vi "soundIn_out.vi"() -> ()   [LabVIEW 2014]
uses:
  <vilib>/sound2/lvsound2.llb/Sound File Info (path).vi
  <vilib>/measure/NI_MAPro.lvlib
  <vilib>/measure/maspectr.llb/FFT Power Spectrum and PSD for 1 Chan.vi
  <vilib>/Math Plots/3D Math Plots/3D Scatter/3D Scatter Datatype/3D Scatter Datatype.lvclass
  <vilib>/Math Plots/3D Math Plots/3D Scatter/3D Scatter Datatype/Public/Plot Helper (Vector).vi
  <vilib>/imath/engines/lvmath2/RunTimeEngine/Managers/WorkSpace/UID Generator.vi
  <vilib>/imath/engines/lvmath2/RunTimeEngine/BuiltInFunctions/length/NIMS_length(GV).vi
  <vilib>/imath/engines/lvmath2/RunTimeEngine/RangeToken/NIMS_Range.vi
  <vilib>/imathl/engines/lvmath/Functions/Error Handling/Create Error.vi
  <vilib>/imath/engines/lvmath2/RunTimeEngine/LocalVariableDefStatement/MC_LocalVariableDefStatement_Display.vi
  <vilib>/imath/engines/lvmath2/RunTimeEngine/RunTimeType/NIMS_RunTimeType_From StrictType (excl LVString).vi
  <vilib>/imath/engines/lvmath2/RunTimeEngine/BuiltInFunctions/ones/NIMS_M=ones(I32).vi
  <vilib>/imath/engines/lvmath2/RunTimeEngine/IndexRead/NIMS M($,S).vi
  <vilib>/imath/engines/lvmath2/RunTimeEngine/RunTimeType/NIMS_RunTimeType_Set Source Original Bool.vi
  <vilib>/imath/engines/lvmath2/RunTimeEngine/Managers/SymbolTable/Clear UID.vi
  <vilib>/imath/engines/lvmath2/RunTimeEngine/NodeEndStatement/NIMS_NodeEndStatement_Output.vi
  <vilib>/imath/engines/lvmath2/RunTimeEngine/ErrorHandling/NIMS_Finalize Error.vi
  <vilib>/sound2/lvsound2.llb/Sound Data Format.ctl
  <vilib>/Math Plots/3D Math Plots/3D Scatter/3D Scatter XCtrl/3D Scatter.xctl
panel:
  out "Time Dependent Power Spectrum":refnum<class "3D Plot Datatype.lvclass">[](xcontrol)
  in  "Play Output":bool
  out "Frequency Power Spectrum":cluster{"f0":dbl, "df":dbl, "magnitude":dbl[]}(graph)={"f0"=0.0, "df"=0.3333333333333333, "magnitude"=array[4500 elements]}
  out "Sound Format: File 2":T1={"sample rate (S/s)"=3000.0, "number of channels"=1, "bits per sample"=16}
  out "Input Audio 2 Waveform":waveform(dbl)(graph)={"t0"=timestamp(0 s since 1904-01-01), "dt"=0.0003333333333333333, "Y"=array[9000 elements]}
  in  "Audio File 2 Path":path=path "C:/Users/jjb22/Documents/GitHub/434_Final_Project/audio_out0.wav"
  in  "Output File Path":path=path "C:/Users/jjb22/Documents/GitHub/434_Final_Project/audio_out1.wav"
  out "Mixed Output Audio Waveform":waveform(dbl)(graph)={"t0"=timestamp(0 s since 1904-01-01), "dt"=0.0003333333333333333, "Y"=array[9000 elements]}
  out "Sound Format: File 1":T1={"sample rate (S/s)"=3000.0, "number of channels"=1, "bits per sample"=16}
  out "Input Audio 1 Waveform":waveform(dbl)(graph)={"t0"=timestamp(0 s since 1904-01-01), "dt"=0.0003333333333333333, "Y"=array[9000 elements]}
  in  "Audio File 1 Path":path=path "C:/Users/jjb22/Documents/GitHub/434_Final_Project/audio_out.wav"
  # "File Name: soundIn_out.vi\nAuthored: Josh Reyes & Josh Borgman\n\nThis VI takes in two audio files and mixes them and normalizes the signal. Optional playback of the mixed output. The power spectrum is computed an ploted below to help the user visualize the audio content."
  # "The plots below use a FFT to compute the power spectrum of the mixed audio signal. The 3D scatter plot displays the power spectrum of 1 second clips  to better visualize the frequency content distribution of the mix signal. The Frequency Power Spectrum displays the power spectrum of the entire waveform."
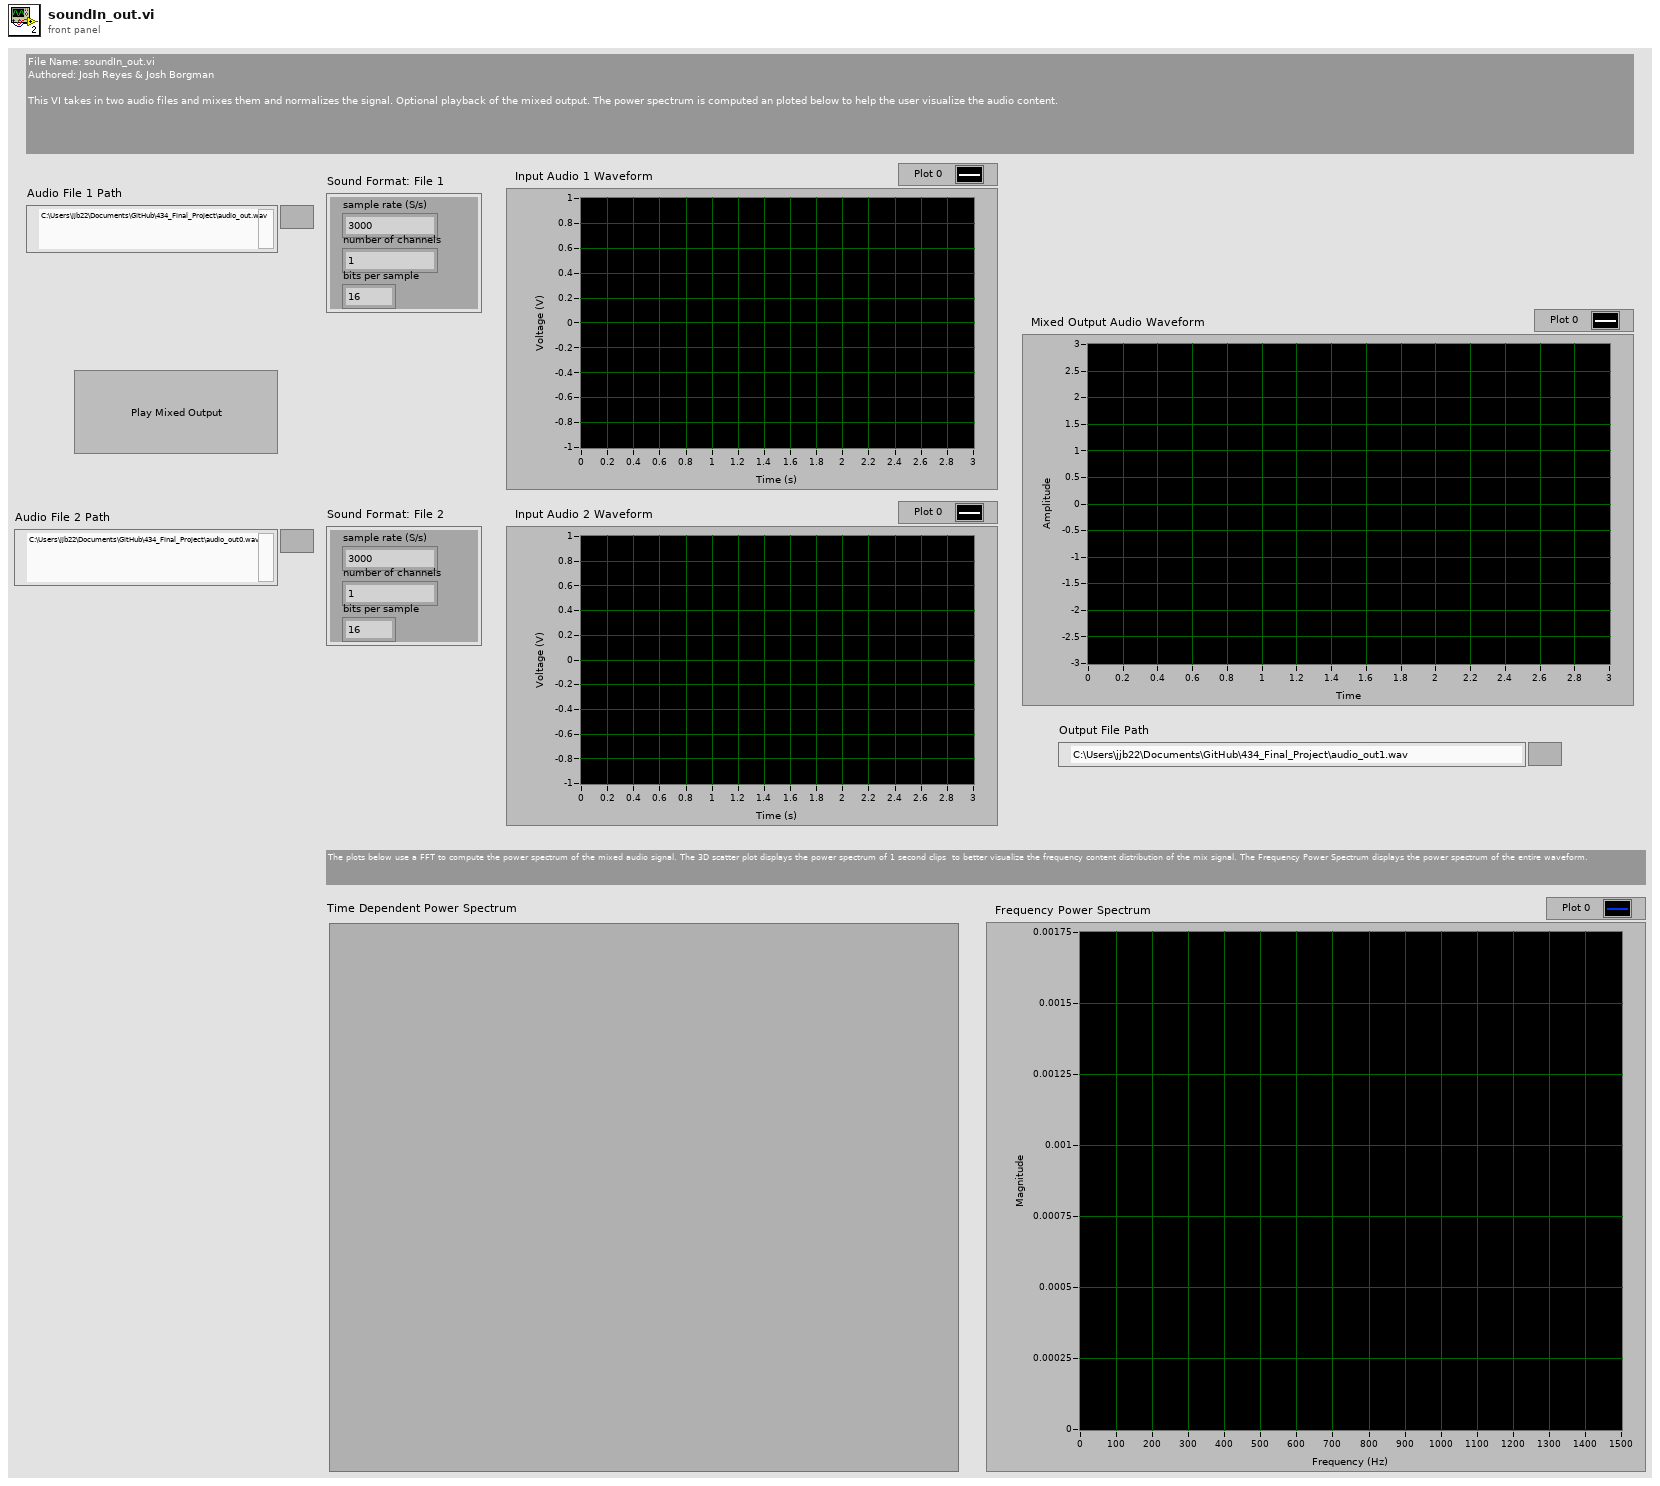
[diagram p1: front panel]
types:
  T1 = typedef "Sound Data Format.ctl" = cluster{"sample rate (S/s)":dbl, "number of channels":i32, "bits per sample":i32}
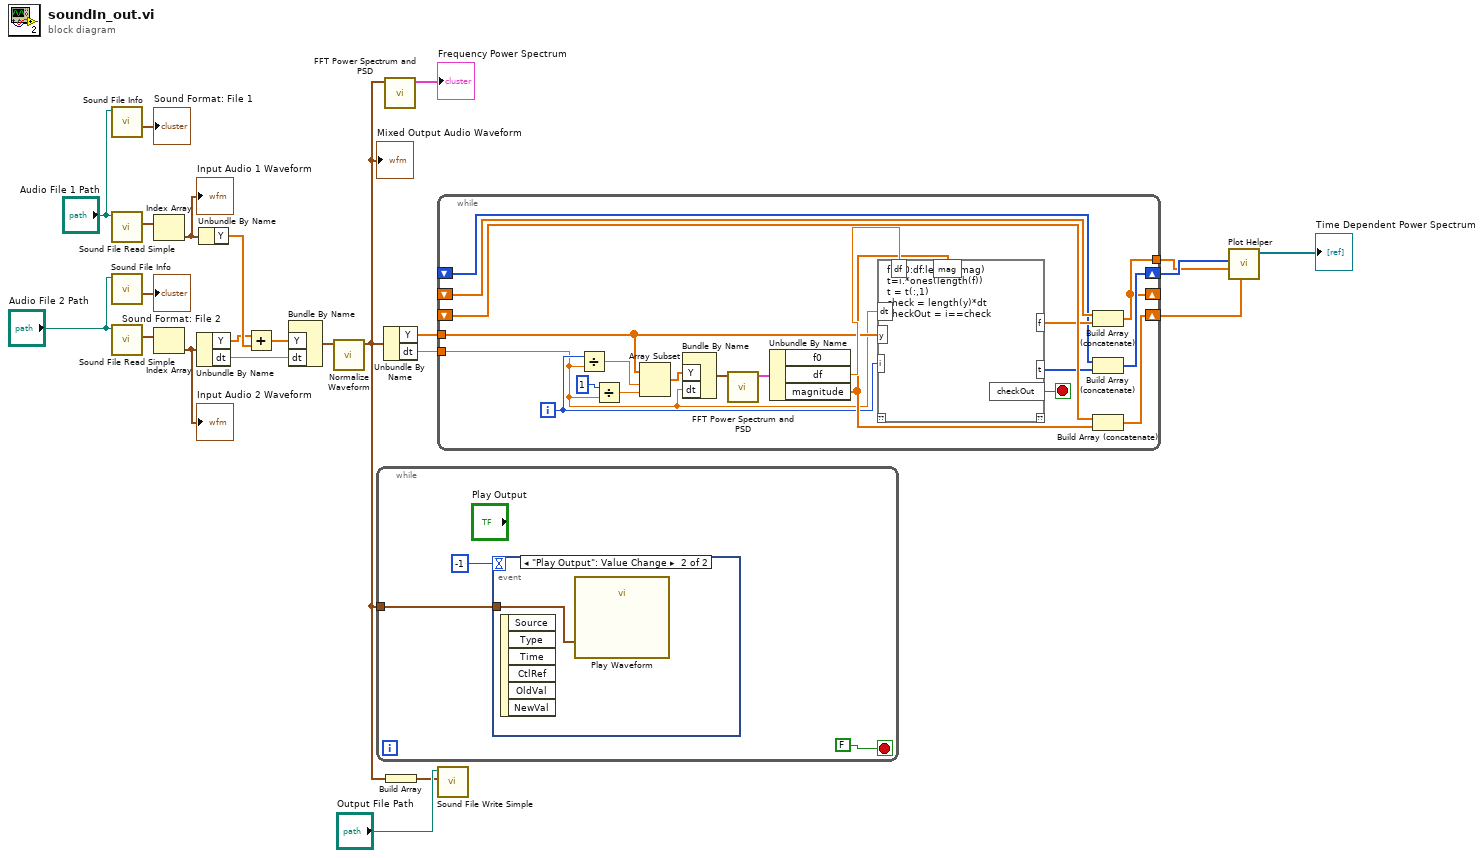
[diagram p0: block diagram]
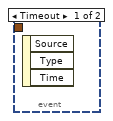
[diagram p2: hidden frame]
diagram:
  n1 = call-poly <vilib>:"Sound File Info.vi"("path"="Audio File 1 Path") -> ("sound format"=→"Sound Format: File 1":T1)  [unwired: 7 in, 3 out]
  n2 = call <vilib>:"Sound File Read Simple.vi"("path"="Audio File 1 Path") -> ("data"=w23:waveform(dbl)[])  [unwired: 7 in, 3 out]
  n3 = call-poly <vilib>:"Sound File Info.vi"("path"="Audio File 2 Path") -> ("sound format"=→"Sound Format: File 2":T1)  [unwired: 7 in, 3 out]
  n4 = call <vilib>:"Sound File Read Simple.vi"("path"="Audio File 2 Path") -> ("data"=w18:waveform(dbl)[])  [unwired: 7 in, 3 out]
  n5 = Index Array(array=w23) -> (element=w22:waveform(dbl))  [unwired: 1 in]
  "Input Audio 1 Waveform" <- w22
  n6 = Index Array(array=w18) -> (element=w17:waveform(dbl))  [unwired: 1 in]
  "Input Audio 2 Waveform" <- w17
  n7 = Unbundle By Name(w17) -> ("Y"=w10:dbl[], "dt"=w9:dbl)
  n8 = Unbundle By Name(w22) -> ("Y"=w13:dbl[])
  n9 = Add(x=w10, y=w13) -> (x+y=w14:dbl[])
  n10 = Bundle By Name("Y"=w14, "dt"=w9) -> (w11:waveform(dbl))  [unwired: 1 in]
  n11 = call <vilib>:"Normalize Waveform.vi"("waveform in"=w11) -> ("normalized waveform"=w7:waveform(dbl))  [unwired: 7 in, 3 out]
  "Mixed Output Audio Waveform" <- w7
  n12 = while {
    tunnel: w7 -> [w25]
    stop <- FALSE stop-if-true
    n13 = event shown="[1] \"Play Output\": Value Change" {
      selector: _ -> [_ _]
      dyn-events: _ -> [_ _]
      timeout: -1 -> [_ _]
      tunnel: w25 -> [_ w27]
      event Timeout {
        n14 = event-data() -> ()  [unwired: 1 in, 3 out]
      }
      event "Play Output": Value Change {
        n15 = event-data() -> ()  [unwired: 1 in, 6 out]
        n16 = call "Play Waveform"("Data"=w27) -> ()  [unwired: 18 in, 1 out]
      }
    }
  }
  n17 = Unbundle By Name(w7) -> ("Y"=w6:dbl[], "dt"=w5:dbl)
  n18 = call-poly <vilib>:"FFT Power Spectrum and PSD.vi"("time signal"=w7) -> ("Power Spectrum / PSD"=→"Frequency Power Spectrum":cluster{"f0":dbl, "df":dbl, "magnitude":dbl[]})  [unwired: 7 in, 3 out]
  n19 = Build Array(w7) -> (w12:waveform(dbl)[])
  n20 = while {
    tunnel: w6 -> [w30]
    tunnel: w5 -> [w29]
    shift-right: [w38] -> w1
    shift-left: _ -> [w40]
    shift-right: [w31] -> _
    shift-left: _ -> [w36]
    shift-right: [w32] -> w3
    shift-left: _ -> [w33]
    tunnel: [w31] -> w2
    i -> [w35]
    stop <- w28 stop-if-true
    n21 = Divide(x=w35, y=w29) -> (x/y=w46:dbl)
    n22 = Divide(x=1, y=w29) -> (x/y=w45:dbl)
    n23 = Array Subset(array=w30, index=w46, length=w45) -> (w43:dbl[])
    n24 = Bundle By Name("Y"=w43, "dt"=w29) -> (w47:waveform(dbl))  [unwired: 1 in]
    n25 = call-poly <vilib>:"FFT Power Spectrum and PSD.vi"("time signal"=w47) -> ("Power Spectrum / PSD"=w42:cluster{"f0":dbl, "df":dbl, "magnitude":dbl[]})  [unwired: 7 in, 3 out]
    n26 = Unbundle By Name(w42) -> ("df"=w41:dbl, "magnitude"=w39:dbl[])  [unwired: 1 out]
    n27 = mathscript code="f = 0:df:length(mag)\nt=i.*ones(length(f))\nt = t(:,1)\ncheck = length(y)*dt\ncheckOut = i==check"("df"=w41, "mag"=w39, "i"=w35, "y"=w30, "dt"=w29) -> ("f"=w37:dbl[], "t"=w34:i32[], "checkOut"=w28:bool)  [unwired: 1 in, 1 out]
    n28 = Build Array (concatenate)(w36, w37) -> (w31:dbl[])
    n29 = Build Array (concatenate)(w33, w34) -> (w32:i32[])
    n30 = Build Array (concatenate)(w40, w39) -> (w38:dbl[])
  }
  n31 = call <vilib>:"Sound File Write Simple.vi"("data"=w12, "path"="Output File Path") -> ()  [unwired: 8 in, 2 out]
  n32 = call-poly <vilib>:"Plot Helper.vi"("z vector"=w1, "y vector"=w2, "x vector"=w3) -> ("3D Plot lvclass Array out"=→"Time Dependent Power Spectrum":refnum<class "3D Plot Datatype.lvclass">[])  [unwired: 3 in, 5 out]
